vi "R1GetSignals.vi"(7 "LabVIEW Web Service Request":refnum<class "Web Request.lvclass">) -> (3 "R1 Signal Status":T1 {"NH4 ISE"."NH4 ISE Signal"."Steady State?" items=["False", "True", "NaN", ""]; "Na ISE"."Na ISE Signal"."Steady State?" items=["False", "True", "NaN", ""]; "K ISE"."K ISE Signal"."Steady State?" items=["False", "True", "NaN", ""]})   [LabVIEW 2016]
uses:
  R1Controls/R7Signal_Status.ctl
  Controls/ISE_CF.ctl
  Controls/Tri State Control.ctl
  <vilib>/wsapi/Web Request.lvclass
panel:
  # "Use the Web Service Request input terminal to call the VIs on the Web Services palette. Do not remove it from the connector pane unless you don't need access to the palette."
  # "Each additional control wired to the connector pane will be available as an input in the URL. To include an indicator in terminal-mode output (the default setting), it must also be wired to the connector pane."
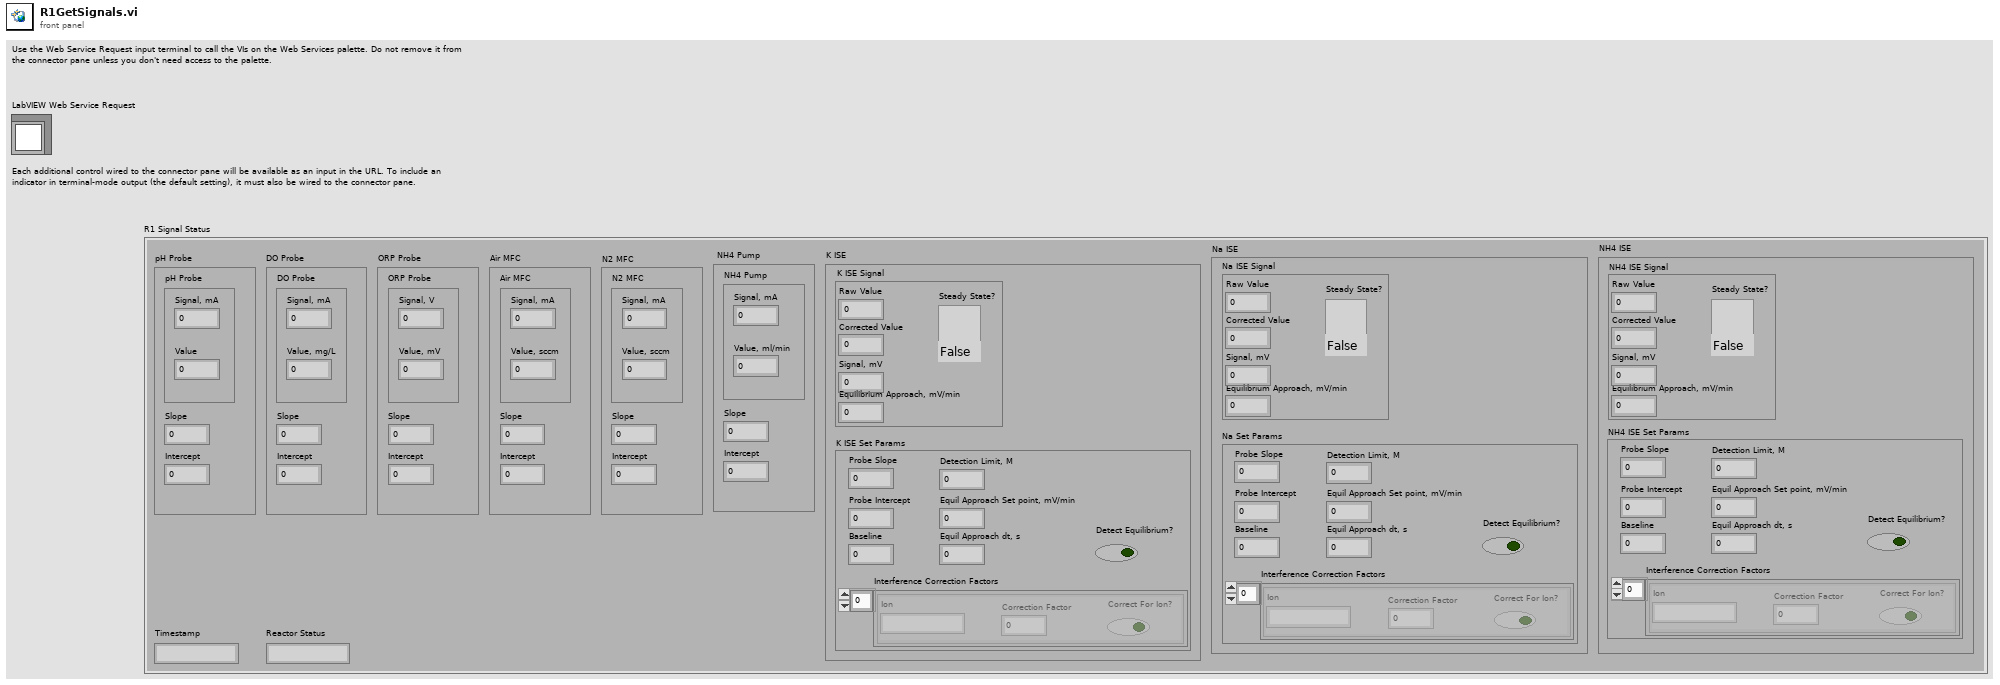
[diagram p1: front panel]
types:
  T1 = typedef "R7Signal_Status.ctl" = cluster{"Timestamp":string, "Reactor Status":string, "pH Probe":cluster{"Slope":dbl, "Intercept":dbl, "pH Probe":cluster{"Signal, mA":dbl, "Value":dbl}}, "DO Probe":cluster{"Slope":dbl, "Intercept":dbl, "DO Probe":cluster{"Signal, mA":dbl, "Value, mg/L":dbl}}, "ORP Probe":cluster{"Slope":dbl, "Intercept":dbl, "ORP Probe":cluster{"Signal, V":dbl, "Value, mV":dbl}}, "Air MFC":cluster{"Slope":dbl, "Intercept":dbl, "Air MFC":cluster{"Signal, mA":dbl, "Value, sccm":dbl}}, "N2 MFC":cluster{"Slope":dbl, "Intercept":dbl, "N2 MFC":cluster{"Signal, mA":dbl, "Value, sccm":dbl}}, "K ISE":cluster{"K ISE Signal ":cluster{"Raw Value":dbl, "Corrected Value":dbl, "Signal, mV":dbl, "Equilibrium Approach, mV/min":dbl, "Steady State?":T2}, "K ISE Set Params":cluster{"Equil Approach Set point, mV/min":dbl, "Equil Approach dt, s":dbl, "Interference Correction Factors":T3[], "Detect Equilibrium?":bool, "Probe Intercept":dbl, "Probe Slope":dbl, "Baseline":dbl, "Detection Limit, M":dbl}}, "Na ISE":cluster{"Na ISE Signal ":cluster{"Raw Value":dbl, "Corrected Value":dbl, "Signal, mV":dbl, "Equilibrium Approach, mV/min":dbl, "Steady State?":T2}, "Na Set Params":cluster{"Equil Approach Set point, mV/min":dbl, "Equil Approach dt, s":dbl, "Interference Correction Factors":T3[], "Detect Equilibrium?":bool, "Probe Intercept":dbl, "Probe Slope":dbl, "Baseline":dbl, "Detection Limit, M":dbl}}, "NH4 ISE":cluster{"NH4 ISE Signal ":cluster{"Raw Value":dbl, "Corrected Value":dbl, "Signal, mV":dbl, "Equilibrium Approach, mV/min":dbl, "Steady State?":T2}, "NH4 ISE Set Params":cluster{"Equil Approach Set point, mV/min":dbl, "Equil Approach dt, s":dbl, "Interference Correction Factors":T3[], "Detect Equilibrium?":bool, "Probe Intercept":dbl, "Probe Slope":dbl, "Baseline":dbl, "Detection Limit, M":dbl}}, " NH4 Pump":cluster{"Slope":dbl, "Intercept":dbl, "NH4 Pump":cluster{"Signal, mA":dbl, "Value, ml/min":dbl}}}
  T2 = typedef "Tri State Control.ctl" = u16
  T3 = typedef "ISE_CF.ctl" = cluster{"Correction Factor":dbl, "Ion":string, "Correct For Ion?":bool}
  T4 = cluster{"Equil Approach Set point, mV/min":dbl, "Equil Approach dt, s":dbl, "Interference Correction Factors":T3[], "Detect Equilibrium?":bool, "Probe Intercept":dbl, "Probe Slope":dbl, "Baseline":dbl, "Detection Limit, M":dbl}
  T5 = cluster{"Signal, mA":dbl, "Value, UNITS HERE":dbl}
  T6 = cluster{"Raw Value":dbl, "Corrected Value":dbl, "Signal, mV":dbl, "Equilibrium Approach, mV/min":dbl, "Steady State?":T2}
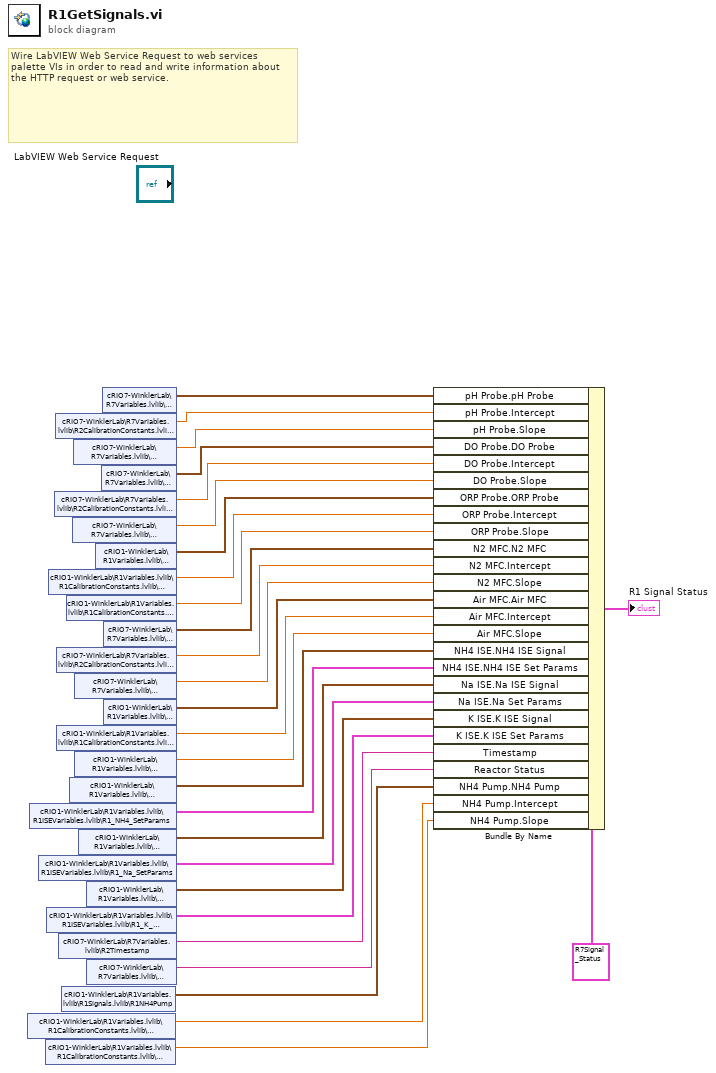
[diagram p0: block diagram]
diagram:
  # "Wire LabVIEW Web Service Request to web services palette VIs in order to read and write information about the HTTP request or web service."
  n1 = shared-variable "cRIO1-WinklerLab\\R1Variables.lvlib\\R1CalibrationConstants.lvlib\\NH4PumpIntercept"() -> (w2:dbl)  [unwired: 1 in, 1 out]
  n2 = shared-variable "cRIO1-WinklerLab\\R1Variables.lvlib\\R1ISEVariables.lvlib\\R1_NH4_SetParams"() -> (w4:T4)  [unwired: 1 in, 1 out]
  n3 = shared-variable "cRIO1-WinklerLab\\R1Variables.lvlib\\R1ISEVariables.lvlib\\R1_Na_SetParams"() -> (w6:T4)  [unwired: 1 in, 1 out]
  n4 = shared-variable "cRIO1-WinklerLab\\R1Variables.lvlib\\R1CalibrationConstants.lvlib\\NH4PumpSlope"() -> (w3:dbl)  [unwired: 1 in, 1 out]
  n5 = shared-variable "cRIO1-WinklerLab\\R1Variables.lvlib\\R1ISEVariables.lvlib\\R1_K_SetParams"() -> (w8:T4)  [unwired: 1 in, 1 out]
  n6 = shared-variable "cRIO1-WinklerLab\\R1Variables.lvlib\\R1CalibrationConstants.lvlib\\R1ORPIntercept"() -> (w19:dbl)  [unwired: 1 in, 1 out]
  n7 = shared-variable "cRIO7-WinklerLab\\R7Variables.lvlib\\R2CalibrationConstants.lvlib\\R2DOIntercept"() -> (w22:dbl)  [unwired: 1 in, 1 out]
  n8 = shared-variable "cRIO7-WinklerLab\\R7Variables.lvlib\\R2CalibrationConstants.lvlib\\R2pHIntercept"() -> (w25:dbl)  [unwired: 1 in, 1 out]
  n9 = shared-variable "cRIO7-WinklerLab\\R7Variables.lvlib\\R2CalibrationConstants.lvlib\\R2N2Intercept"() -> (w16:dbl)  [unwired: 1 in, 1 out]
  n10 = shared-variable "cRIO1-WinklerLab\\R1Variables.lvlib\\R1CalibrationConstants.lvlib\\R1AirIntercept"() -> (w13:dbl)  [unwired: 1 in, 1 out]
  n11 = shared-variable "cRIO7-WinklerLab\\R7Variables.lvlib\\R2Timestamp"() -> (w9:string)  [unwired: 1 in, 1 out]
  n12 = shared-variable "cRIO1-WinklerLab\\R1Variables.lvlib\\R1Signals.lvlib\\R1NH4Pump"() -> (w1:T5)  [unwired: 1 in, 1 out]
  n13 = shared-variable "cRIO1-WinklerLab\\R1Variables.lvlib\\R1CalibrationConstants.lvlib\\R1ORPSlope"() -> (w18:dbl)  [unwired: 1 in, 1 out]
  n14 = shared-variable "cRIO1-WinklerLab\\R1Variables.lvlib\\R1ISEVariables.lvlib\\R1_NH4_ISE"() -> (w11:T6)  [unwired: 1 in, 1 out]
  n15 = shared-variable "cRIO7-WinklerLab\\R7Variables.lvlib\\R2CalibrationConstants.lvlib\\R2DOSlope"() -> (w21:dbl)  [unwired: 1 in, 1 out]
  n16 = shared-variable "cRIO7-WinklerLab\\R7Variables.lvlib\\R2CalibrationConstants.lvlib\\R2pHSlope"() -> (w24:dbl)  [unwired: 1 in, 1 out]
  n17 = shared-variable "cRIO7-WinklerLab\\R7Variables.lvlib\\R2CalibrationConstants.lvlib\\R2N2Slope"() -> (w15:dbl)  [unwired: 1 in, 1 out]
  n18 = shared-variable "cRIO1-WinklerLab\\R1Variables.lvlib\\R1CalibrationConstants.lvlib\\R1AirSlope"() -> (w12:dbl)  [unwired: 1 in, 1 out]
  n19 = shared-variable "cRIO1-WinklerLab\\R1Variables.lvlib\\R1ISEVariables.lvlib\\R1_Na_ISE"() -> (w5:T6)  [unwired: 1 in, 1 out]
  n20 = shared-variable "cRIO1-WinklerLab\\R1Variables.lvlib\\R1ISEVariables.lvlib\\R1_K_ISE"() -> (w7:T6)  [unwired: 1 in, 1 out]
  n21 = shared-variable "cRIO7-WinklerLab\\R7Variables.lvlib\\R2Status"() -> (w10:string)  [unwired: 1 in, 1 out]
  n22 = shared-variable "cRIO1-WinklerLab\\R1Variables.lvlib\\R1Signals.lvlib\\R1ORP"() -> (w20:T5)  [unwired: 1 in, 1 out]
  n23 = shared-variable "cRIO7-WinklerLab\\R7Variables.lvlib\\R2Signals.lvlib\\R1DO"() -> (w23:cluster{"Signal":dbl, "Value":dbl})  [unwired: 1 in, 1 out]
  n24 = shared-variable "cRIO7-WinklerLab\\R7Variables.lvlib\\R2Signals.lvlib\\R1pH"() -> (w27:cluster{"Signal":dbl, "Value":dbl})  [unwired: 1 in, 1 out]
  n25 = shared-variable "cRIO7-WinklerLab\\R7Variables.lvlib\\R2Signals.lvlib\\R1N2"() -> (w17:cluster{"Signal":dbl, "Value":dbl})  [unwired: 1 in, 1 out]
  n26 = shared-variable "cRIO1-WinklerLab\\R1Variables.lvlib\\R1Signals.lvlib\\R1Air"() -> (w14:T5)  [unwired: 1 in, 1 out]
  n27 = Bundle By Name(cluster=T1 {"Timestamp"="", "Reactor Status"="", "pH Probe"={"Slope"=0.0, "Intercept"=0.0, "pH Probe"={"Signal, mA"=0.0, "Value"=0.0}}, "DO Probe"={"Slope"=0.0, "Intercept"=0.0, "DO Probe"={"Signal, mA"=0.0, "Value, mg/L"=0.0}}, "ORP Probe"={"Slope"=0.0, "Intercept"=0.0, "ORP Probe"={"Signal, V"=0.0, "Value, mV"=0.0}}, "Air MFC"={"Slope"=0.0, "Intercept"=0.0, "Air MFC"={"Signal, mA"=0.0, "Value, sccm"=0.0}}, "N2 MFC"={"Slope"=0.0, "Intercept"=0.0, "N2 MFC"={"Signal, mA"=0.0, "Value, sccm"=0.0}}, "K ISE"={"K ISE Signal "={"Raw Value"=0.0, "Corrected Value"=0.0, "Signal, mV"=0.0, "Equilibrium Approach, mV/min"=0.0, "Steady State?"=0}, "K ISE Set Params"={"Equil Approach Set point, mV/min"=0.0, "Equil Approach dt, s"=0.0, "Interference Correction Factors"=[], "Detect Equilibrium?"=FALSE, "Probe Intercept"=0.0, "Probe Slope"=0.0, "Baseline"=0.0, "Detection Limit, M"=0.0}}, "Na ISE"={"Na ISE Signal "={"Raw Value"=0.0, "Corrected Value"=0.0, "Signal, mV"=0.0, "Equilibrium Approach, mV/min"=0.0, "Steady State?"=0}, "Na Set Params"={"Equil Approach Set point, mV/min"=0.0, "Equil Approach dt, s"=0.0, "Interference Correction Factors"=[], "Detect Equilibrium?"=FALSE, "Probe Intercept"=0.0, "Probe Slope"=0.0, "Baseline"=0.0, "Detection Limit, M"=0.0}}, "NH4 ISE"={"NH4 ISE Signal "={"Raw Value"=0.0, "Corrected Value"=0.0, "Signal, mV"=0.0, "Equilibrium Approach, mV/min"=0.0, "Steady State?"=0}, "NH4 ISE Set Params"={"Equil Approach Set point, mV/min"=0.0, "Equil Approach dt, s"=0.0, "Interference Correction Factors"=[], "Detect Equilibrium?"=FALSE, "Probe Intercept"=0.0, "Probe Slope"=0.0, "Baseline"=0.0, "Detection Limit, M"=0.0}}, " NH4 Pump"={"Slope"=0.0, "Intercept"=0.0, "NH4 Pump"={"Signal, mA"=0.0, "Value, ml/min"=0.0}}} ("Signal Status"), "pH Probe.pH Probe"=w27, "pH Probe.Intercept"=w25, "pH Probe.Slope"=w24, "DO Probe.DO Probe"=w23, "DO Probe.Intercept"=w22, "DO Probe.Slope"=w21, "ORP Probe.ORP Probe"=w20, "ORP Probe.Intercept"=w19, "ORP Probe.Slope"=w18, "N2 MFC.N2 MFC"=w17, "N2 MFC.Intercept"=w16, "N2 MFC.Slope"=w15, "Air MFC.Air MFC"=w14, "Air MFC.Intercept"=w13, "Air MFC.Slope"=w12, "NH4 ISE.NH4 ISE Signal"=w11, "NH4 ISE.NH4 ISE Set Params"=w4, "Na ISE.Na ISE Signal"=w5, "Na ISE.Na Set Params"=w6, "K ISE.K ISE Signal"=w7, "K ISE.K ISE Set Params"=w8, "Timestamp"=w9, "Reactor Status"=w10, "NH4 Pump.NH4 Pump"=w1, "NH4 Pump.Intercept"=w2, "NH4 Pump.Slope"=w3) -> (→"R1 Signal Status":T1)
